vi "installer_compress.vi"(6 "distribution_folder":path, 8 "error in (no error)":errorcluster, 11 "build_specifications":T1) -> (0 "error out":errorcluster)   [LabVIEW 2015, in "lv-builder-default.lvlib"]
uses:
  lv-builder-default.lvlib
  lv-build/public/_controls/build_specification.ctl
  lv-build/public/_controls/build_type.ctl
  <userlib>/antonio-alexander/lv-bin-7zip/public/api/v1/advanced/compress_exe.vi
  <userlib>/antonio-alexander/lv-bin-7zip/public/api/v1/v1.lvlib
  lv-build/lv-build.lvlib
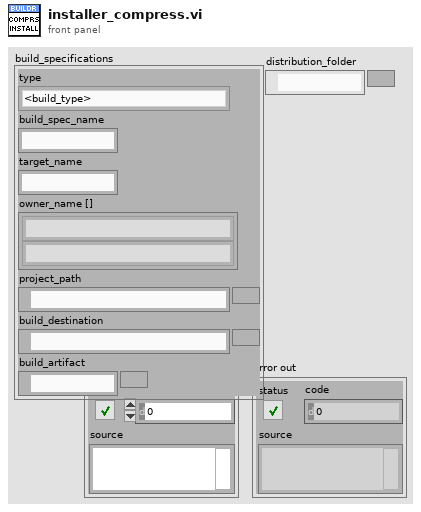
[diagram p1: front panel]
types:
  T1 = typedef "lv-build.lvlib/build_specification.ctl" = cluster{"type":T2, "build_spec_name":string, "target_name":string, "owner_name []":string[], "project_path":path, "build_destination":path, "build_artifact":path}
  T2 = typedef "lv-build.lvlib/build_type.ctl" = enum16{"<build_type>", "application_pc", "application_rt", "installer", "llb", "lvlibp", "zip", "fpga", "<null>"}
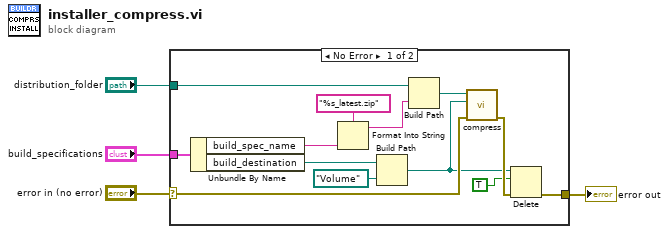
[diagram p0: block diagram]
diagram:
  n1 = case shown="No Error" "error in (no error)" {
    selector: "error in (no error)" -> [w9 w18]
    tunnel: "build_specifications" -> [w17 _]
    tunnel: [w7 w18] -> w2
    tunnel: "distribution_folder" -> [w11 _]
    frame No Error {
      n2 = Unbundle By Name(w17) -> ("build_spec_name"=w14:string, "build_destination"=w10:path)
      n3 = Format Into String(format string="%s_latest.zip", w14) -> (resulting string=w13:string)  [unwired: 2 in, 1 out]
      n4 = Build Path(base path=w10, name or relative path=path "Volume" ("BuildDestination")) -> (appended path=w6:path)
      n5 = Build Path(base path=w11, name or relative path=w13) -> (appended path=w12:path)
      n6 = call-poly <userlib>:"compress.vi"("error in (no error)"=w9, "files_to_add"=w6, "archive_path in"=w12) -> ("error out"=w8:errorcluster)  [unwired: 7 in, 1 out]
      n7 = Delete(path (use dialog)=w6, entire hierarchy (F)=TRUE, error in=w8) -> (error out=w7:errorcluster)  [unwired: 2 in, 2 out]
    }
    frame Error {
    }
  }
  "error out" <- w2
